vi "Initialization.vi"(8 "error in (no error)":errorcluster, 11 "TELEDINE_LECROY in":refnum<class "TELEDINE_LECROY.lvclass">) -> (0 "error out":errorcluster, 3 "TELEDINE_LECROY out":refnum<class "TELEDINE_LECROY.lvclass">)   [LabVIEW 2015, in "TELEDINE_LECROY.lvclass"]
uses:
  TELEDINE_LECROY.lvclass
  GeneralFunctionality/GeneralFunctionality.lvclass/GeneralFunctionality.ctl
  Oscilloscope.lvclass/Oscilloscope.ctl
  Config/Config.lvclass
  LeCroy Wave Series/LeCroy Wave Series.lvlib
  Oscilloscope.lvclass
  GeneralFunctionality/GeneralFunctionality.lvclass
panel:
  in  "Perform Auto Setup?":bool
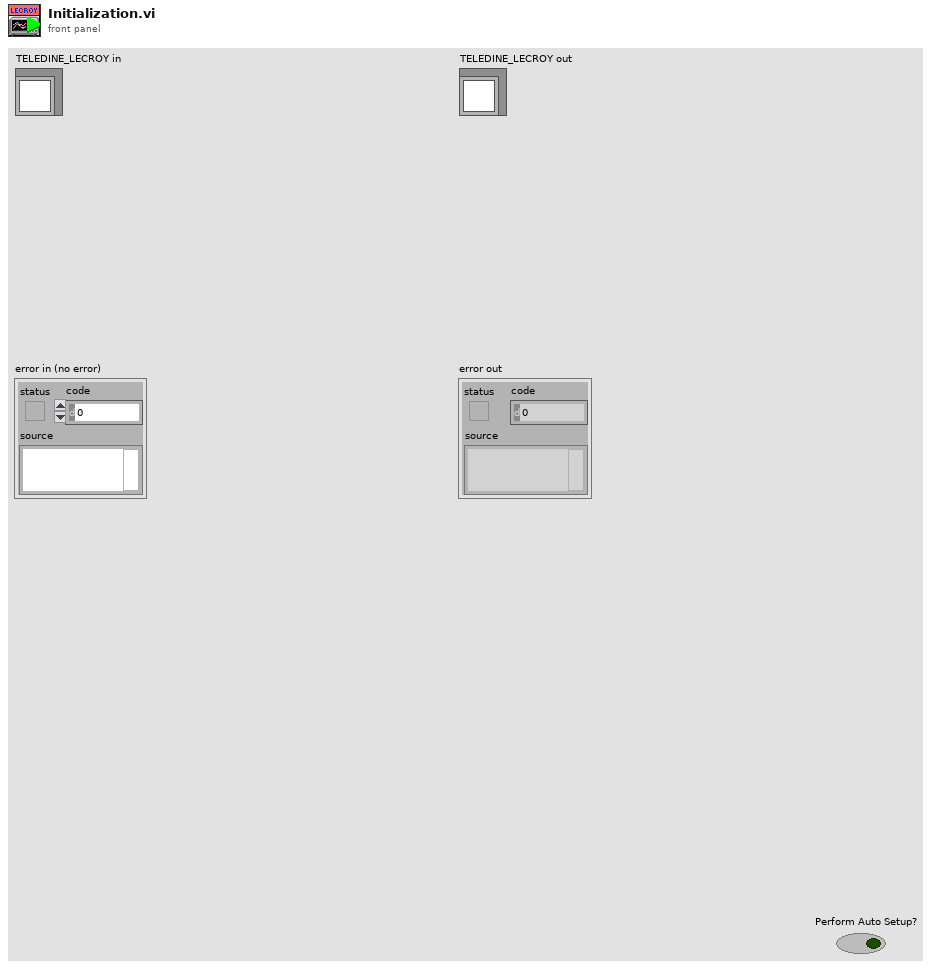
[diagram p1: front panel]
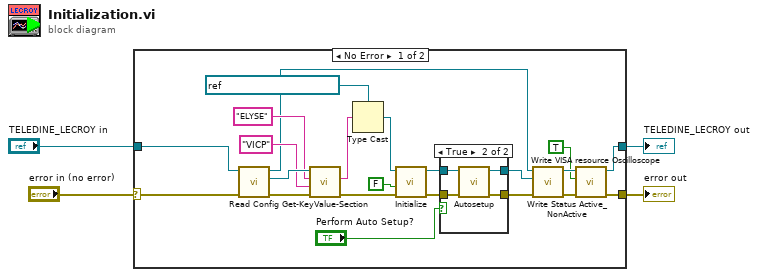
[diagram p0: block diagram]
diagram:
  n1 = case shown="No Error" "error in (no error)" {
    selector: "error in (no error)" -> [w23 w34]
    tunnel: [w8 w34] -> w3
    tunnel: [w9 w33] -> w1
    tunnel: "TELEDINE_LECROY in" -> [w12 w33]
    frame No Error {
      n2 = call "Read Config.vi"("error in (no error)"=w23, "GeneralFunctionality en entrée"=w12) -> ("error out"=w22:errorcluster, "Config.lvclass"=w21:refnum<class "Config.lvclass">, "GeneralFunctionality en sortie"=w16:refnum<class "TELEDINE_LECROY.lvclass">)  [unwired: 7 in]
      n3 = call-dynamic "Get-KeyValue-Section.vi"("error in (no error)"=w22, "Key"="VICP" ("Section"), "Section"="ELYSE", "Config in"=w21) -> ("error out"=w14:errorcluster, "Value"=w18:string)  [unwired: 5 in, 1 out]
      n4 = Type Cast(type=refnum<visa-resource-name> "VICP::129.175.100.26" ("VISA resource name"), x=w18) -> (*(type *) &x=w5:refnum<visa-resource-name>)
      n5 = call "Initialize.vi"("error in (no error)"=w14, "Reset? (T: Yes)"=FALSE, "VISA resource name"=w5) -> ("error out"=w26:errorcluster, "VISA resource name out"=w25:refnum<visa-resource-name>)  [unwired: 7 in]
      n6 = case shown="True" "Perform Auto Setup?" {
        tunnel: w26 -> [w27 w32]
        tunnel: w25 -> [w28 w31]
        tunnel: [w28 w30] -> w13
        tunnel: [w27 w29] -> w15
        frame False {
        }
        frame True {
          n7 = call "Autosetup.vi"("error in (no error)"=w32, "VISA resource name"=w31) -> ("error out"=w29:errorcluster, "VISA resource name out"=w30:refnum<visa-resource-name>)  [unwired: 8 in]
        }
      }
      n8 = call "Write VISA resource Oscilloscope.vi"("error in (no error)"=w15, "VISA resource Oscilloscope"=w13, "Oscilloscope in"=w16) -> ("error out"=w11:errorcluster, "Oscilloscope out"=w10:refnum<class "TELEDINE_LECROY.lvclass">)  [unwired: 7 in]
      n9 = call "Write Status Active_NonActive.vi"("error in (no error)"=w11, "Status Active/NonActive"=TRUE, "GeneralFunctionality in"=w10) -> ("error out"=w8:errorcluster, "GeneralFunctionality out"=w9:refnum<class "TELEDINE_LECROY.lvclass">)  [unwired: 7 in]
    }
    frame Error {
    }
  }
  "error out" <- w3
  "TELEDINE_LECROY out" <- w1
